vi "01 Pretty Plots.vi"() -> ()   [LabVIEW 2019]
uses:
  <userlib>/ME35/Course/_Subs/OpenDiagram/Open_XControl.xctl
panel:
  in  "OpenDiag":refnum<vi>(xcontrol)
  out "XY Graph":cluster{"X":i32[], dbl[]}(graph)
  # "01 Challenge: Pretty Plots\n\nCan you:\n1. make the plot line red (with symbols) on a black background?\n2. label the axes properly?\n3. make the grey part transparent and make the entire VI have a white background?\n4. make the x values twice what they currently are\n5. replace the y value with the sin (y / 10)\n6. generate a new graph that plots two cycles of a sine wave\n7. generate an intensity plot of a sin vs cos wave (Z = Asin(x) + cos(y))"
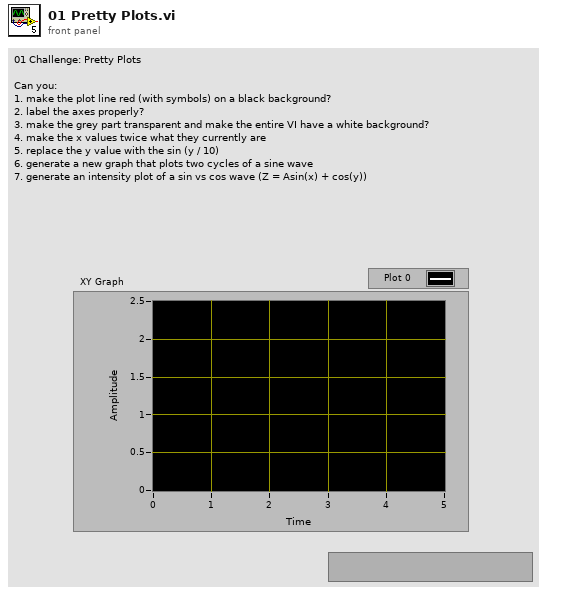
[diagram p1: front panel]
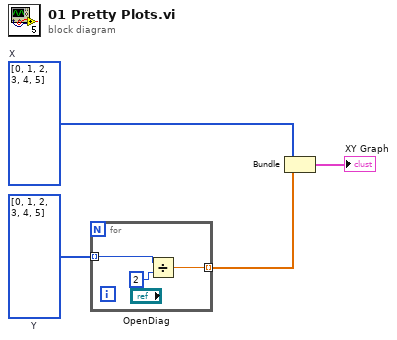
[diagram p0: block diagram]
diagram:
  w4 = i32[] [0, 1, 2, 3, 4, 5]  # Y
  w1 = i32[] [0, 1, 2, 3, 4, 5]  # X
  n1 = for {
    tunnel: w4 -> [w7] mode=indexing
    tunnel: [w5] -> w3 mode=indexing
    # "runs for each element in Y"
    n2 = Divide(x=w7, y=2) -> (x/y=w5:dbl)
  }
  n3 = Bundle("X"=w1, w3) -> (→"XY Graph":cluster{"X":i32[], dbl[]})  [unwired: 1 in]
